vi "AFM_Driver_Manager.CreatePublicEvents.vi"(8 "error in (no error)":errorcluster, 11 "AFM_Driver_Manager in":refnum<class "AFM_Driver_Manager.lvclass">) -> (0 "error out":errorcluster, 3 "AFM_Driver_Manager out":refnum<class "AFM_Driver_Manager.lvclass">)   [LabVIEW 2019, in "AFM_Driver_Manager.lvclass"]
uses:
  AFM_Driver_Manager.lvclass
  AFM_Driver_Manager.lvclass/AFM_Driver_Manager.ctl
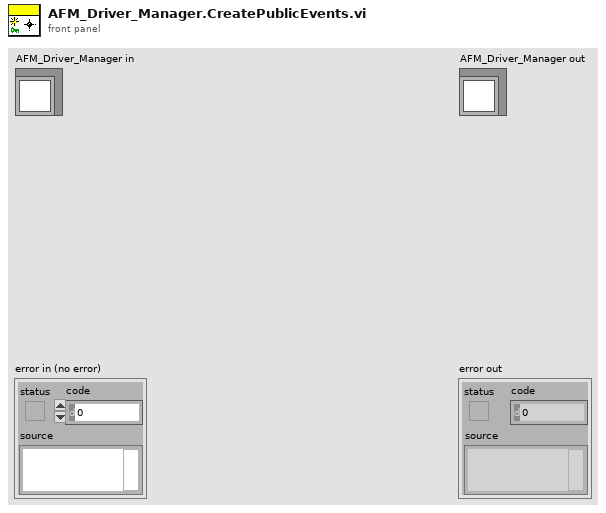
[diagram p1: front panel]
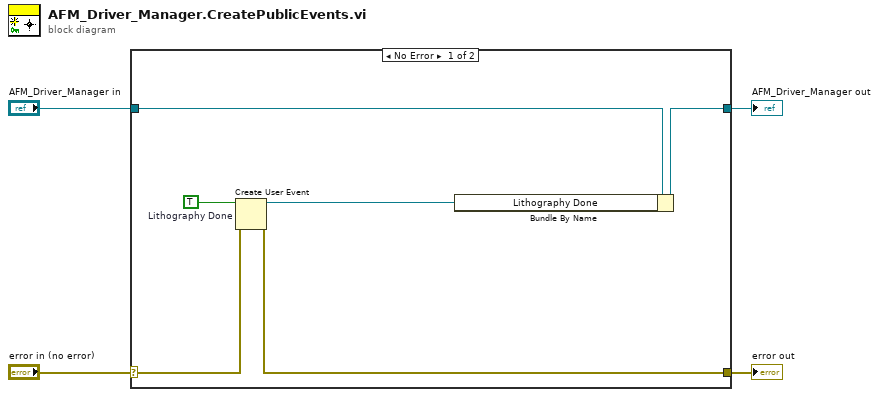
[diagram p0: block diagram]
diagram:
  n1 = case shown="No Error" "error in (no error)" {
    selector: "error in (no error)" -> [w10 w12]
    tunnel: [w9 w12] -> w3
    tunnel: [w8 w11] -> w1
    tunnel: "AFM_Driver_Manager in" -> [w7 w11]
    frame No Error {
      w5 = TRUE  # Lithography Done
      n2 = Create User Event(user event datatype=w5, error in=w10) -> (user event=w6:refnum<user-event>, error out=w9:errorcluster)
      n3 = Bundle By Name(cluster=w7, "Lithography Done"=w6) -> (w8:refnum<class "AFM_Driver_Manager.lvclass">)
    }
    frame Error {
    }
  }
  "error out" <- w3
  "AFM_Driver_Manager out" <- w1
